vi "Manager.vi"   [LabVIEW 2021, in "PluginManager.lvlib"]
uses:
  PluginManager.lvlib
  CIFPluginManager/CIFPluginManager.lvclass
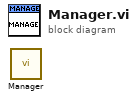
[diagram p0: block diagram]
diagram:
  n1 = call "Manager.vi"() -> ()  [unwired: 12 in]
